vi "Initialize  (MWT) (SubVI).vi"(5 "Min Contour Points":u16=127, 7 "N Spline Points":fxp<+,8,8>=41.0, 8 "REF IN":T5, 10 "Settings File Name":path=path "C:/MWT/Config.ini", 11 "Parameters In":T1={"File REF"={"AVI REF"=refnum, "DBDE REF"=refnum}, "Frame Data"={"Width"=0, "Height"=0, "Frames Per Second"=0, "Codec"=""}, "File Type"="", "Experiment Mode"=enum."Replay", "Movie File Path"=path "D:/Movies Formatted on November 5th 2015/Clip (2) Formatted.raw"}) -> (0 "REF OUT":T5, 3 "Parameters Out":T1={"File REF"={"AVI REF"=refnum, "DBDE REF"=refnum}, "Frame Data"={"Width"=0, "Height"=0, "Frames Per Second"=0, "Codec"=""}, "File Type"="", "Experiment Mode"=enum."Replay", "Movie File Path"=path "D:/Movies Formatted on November 5th 2015/Clip (2) Formatted.raw"}, 4 "Exp. Status":string="Camera Connected", 6 "OK?":bool)   [LabVIEW 2020]
uses:
  Controls (HOST)/REF.ctl
  Controls (HOST)/Image Queue Bundle.ctl
  Controls (HOST)/Data to Disk Bundle.ctl
  Controls (HOST)/File Name Prefix.ctl
  Controls (HOST)/FPGA REF (MWT).ctl
  Controls (HOST)/IMAQ Parameters.ctl
  Controls (HOST)/File REF.ctl
  <vilib>/vision/Avi.llb/IMAQ AVI2 Refnum.ctl
  Controls (HOST)/Experiment Mode.ctl
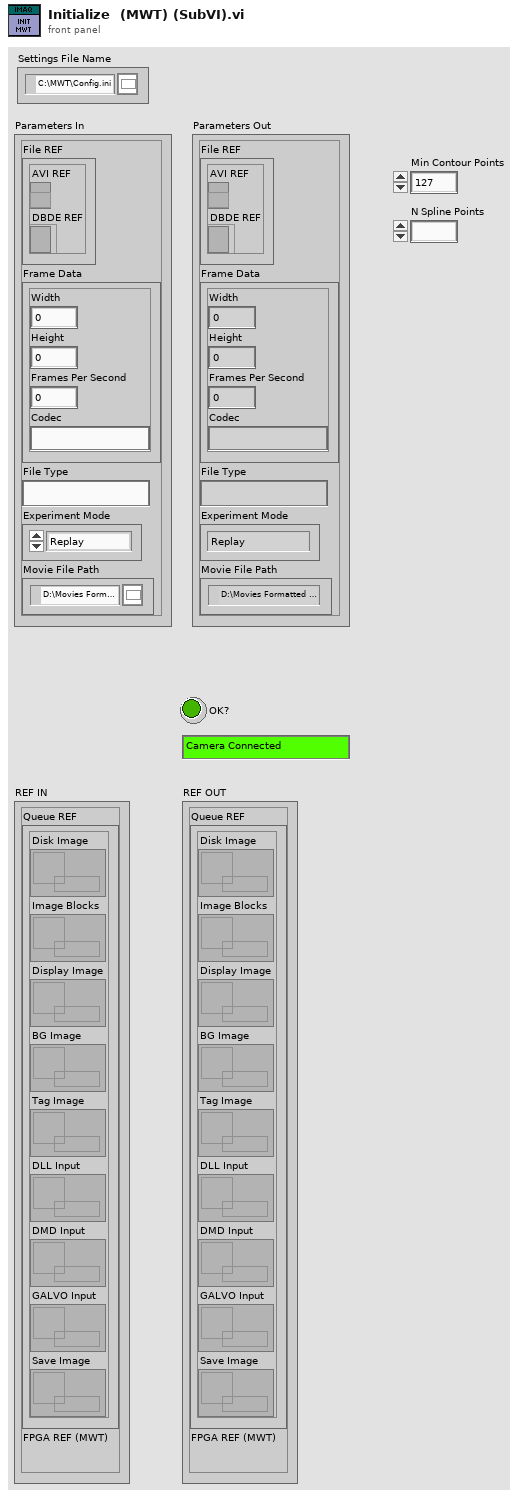
[diagram p1: front panel]
types:
  T1 = typedef "IMAQ Parameters.ctl" = cluster{"File REF":T2, "Frame Data":cluster{"Width":u32, "Height":u32, "Frames Per Second":u32, "Codec":string}, "File Type":string, "Experiment Mode":T4, "Movie File Path":path}
  T2 = typedef "File REF.ctl" = cluster{"AVI REF":T3, "DBDE REF":refnum<file>}
  T3 = typedef "IMAQ AVI2 Refnum.ctl" = refnum<k20>
  T4 = typedef "Experiment Mode.ctl" = enum16{"Live", "Replay"}
  T5 = typedef "REF.ctl" = cluster{"Queue REF":T6, "FPGA REF (MWT)":T7}
  T6 = typedef "Image Queue Bundle.ctl" = cluster{"Disk Image":refnum<queue>, "Image Blocks":refnum<queue>, "Display Image":refnum<queue>, "BG Image":refnum<queue>, "Tag Image":refnum<queue>, "DLL Input":refnum<queue>, "DMD Input":refnum<queue>, "GALVO Input":refnum<queue>, "Save Image":refnum<queue>}
  T7 = typedef "FPGA REF (MWT).ctl" = refnum<k20>
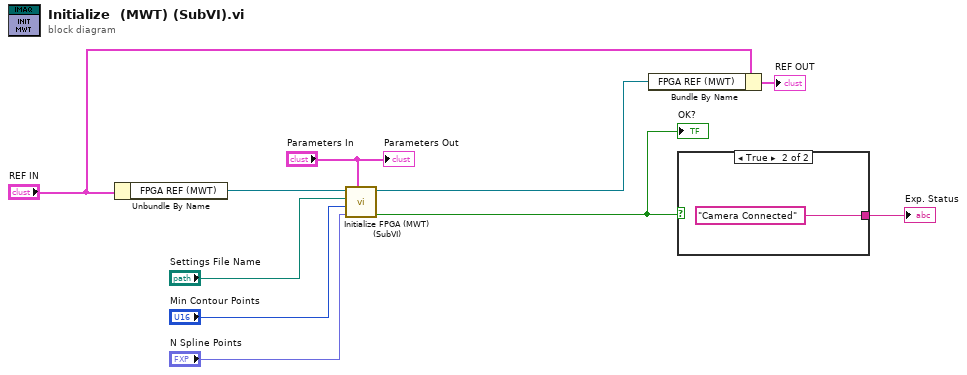
[diagram p0: block diagram]
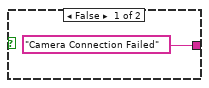
[diagram p2: hidden frame]
diagram:
  n1 = Unbundle By Name("REF IN") -> ("FPGA REF (MWT)"=w10:T7)
  n2 = call "Initialize FPGA (MWT) (SubVI).vi"("Parameters"="Parameters In", "N Spline Points"="N Spline Points", "Min Contour Points"="Min Contour Points", "Settings File Name"="Settings File Name", "FPGA REF (MWT) IN"=w10) -> ("Camera OK?"=w8:bool, "FPGA REF (DBDE) OUT"=w5:T7)  [unwired: 5 in]
  "OK?" <- w8
  n3 = Bundle By Name(cluster="REF IN", "FPGA REF (MWT)"=w5) -> (→"REF OUT":T5)
  n4 = case shown="True" w8 {
    tunnel: ["Camera Connection Failed" "Camera Connected"] -> w9
    frame False {
    }
    frame True {
    }
  }
  "Exp. Status" <- w9
  "Parameters Out" <- "Parameters In"
